vi "niDTS WLAN Rx Test Example.vi"() -> ()   [LabVIEW 2014]
uses:
  Includes/niDTS WLAN INC Type.ctl
  Rx Test/Includes/niDTS WLAN Rx Test INC Results.ctl
  CommLib/Includes/niDTS Comm INC EXE Port Parameters.ctl
  CommLib/Includes/niDTS Comm INC Telnet Port Parameters.ctl
  CommLib/Includes/niDTS Comm INC CLI Login.ctl
  HT Rx Test/Includes/niDTS WLAN HT Rx Test INC HT Parameters.ctl
  Includes/niDTS WLAN INC CH BW HT.ctl
  Includes/niDTS WLAN INC GI.ctl
  Includes/niDTS WLAN INC FEC Coding.ctl
  Rx Test/Includes/niDTS WLAN INC RX Measurement Parameters.ctl
  VHT Rx Test/Includes/niDTS WLAN VHT Rx Test INC Parameters.ctl
  Includes/niDTS WLAN INC CH BW.ctl
  OFDM Rx Test/Includes/niDTS WLAN Rx Test INC OFDM Parameters.ctl
  Includes/niDTS WLAN INC OFDM Data Rate.ctl
  Includes/niDTS WLAN INC CH BW DSSS.ctl
  TestStand/Station/Objects/SystemDutHandle/niDTS SystemDutHandle.lvclass
  niDTS WLAN.lvlib
  Plugins/niBCM4350/niBCM4350.lvlib
  Framework/niDTS Framework.lvlib
  TestStand/niDTS TestStand.lvlib
  Plugins/niBCM4360/niBCM4360.lvlib
  CommLib/niDTS CommLib.lvlib
  Plugins/niBCM4356/niBCM4356.lvlib
panel:
  in  "Socket Index":i32
  in  "System Configuration XML Path":path=path "C:/Users/Public/Documents/National Instruments/WTM 1.0/System Configurations"
  in  "Hardware Manifest XML":path=path "C:/Users/Public/Documents/National Instruments/WTM 1.0/Hardware Manifests"
  in  "Tab Control":enum32{"OFDM", "HT", "VHT"}(tab)=enum."HT"
  in  "OFDM Parameters":T1={"OFDM Data Rate (Mbps)"=enum."54", "Chains"=[TRUE, FALSE, FALSE, FALSE], "Bandwidth (Hz)"=enum."20 MHz", "Channel"=36, "Power (dBm)"=-50.0, "16 symbols"=TRUE, "Payload Length (bytes)"=1500, "Idle Interval (s)"=0.0001, "External Attenuation (dB)"=[2.0, 0.0, 0.0, 0.0], "RX Measurement Parameters"={"Number of Packets"=1000, "MacAddress"="FF:FF:FF:FF:FF:FF"}} {"Idle Interval (s)" format="%_3p"}
  in  "HT Parameters":T5={"MCS Index"=7, "Chains"=[TRUE, FALSE, FALSE, FALSE], "Bandwidth (Hz)"=enum."20 MHz", "Channel"=36, "Power (dBm)"=-45.0, "Guard Interval"=enum."LONG", "FEC Coding"=enum."LDPC", "16 symbols"=TRUE, "Payload Length (bytes)"=1500, "Idle Interval (s)"=5e-05, "External Attenuation (dB)"=[0.0, 0.0, 0.0, 0.0], "RX Measurement Parameters"={"Number of Packets"=1000, "MacAddress"="FF:FF:FF:FF:FF:FF"}} {"Idle Interval (s)" format="%_3p"}
  in  "VHT Parameters":T9={"MCS Index"=7, "N Spatial Streams"=1, "Chains"=[TRUE, FALSE, FALSE, FALSE], "Bandwidth (Hz)"=enum."20 MHz", "Channel"=36, "Power (dBm)"=-45.0, "Guard Interval"=enum."LONG", "FEC Coding"=enum."LDPC", "16 symbols"=TRUE, "Payload Length (bytes)"=1500, "Idle Interval (s)"=2.5e-05, "External Attenuation (dB)"=[0.0, 0.0, 0.0, 0.0], "RX Measurement Parameters"={"Number of Packets"=1000, "MacAddress"="FF:FF:FF:FF:FF:FF"}} {"Idle Interval (s)" format="%_3p"}
  out "error out":errorcluster
  in  "DUT Plugin":enum32{"BCM4360", "BCM4350", "BCM4356"}(tab)=enum."BCM4356"
  in  "Interfaces BCM4350":enum32{".EXE", "Telnet"}(tab)
  in  "General Parameters bcm4350 exe":T12={"WLAN"={"Port Parameters EXE"={"Timeout (s)"=5.0}}} caption="General Parameters"
  in  "Socket Parameters bcm4350 exe":cluster{"WLAN":cluster{"IP Address":string}}={"WLAN"={"IP Address"="192.168.1.1"}} caption="Socket Parameters"
  in  "Socket Parameters bcm4350 telnet":cluster{"WLAN":cluster{"IP Address":string}}={"WLAN"={"IP Address"="192.168.1.1"}} caption="Socket Parameters"
  in  "General Parameters bcm4350 telnet":T15={"WLAN"={"Port Parameters Telnet"={"Bytes to Read"=1000, "Line Separator"="\n", "Port Timeout (ms)"=5000, "Read Mode"=enum."normal", "Write Mode"=enum."normal", "Remote Port"=23}, "CLI Login"={"Do Login"=FALSE, "Login Prompt"="", "Password"="", "User Name"=""}}} caption="General Parameters"
  in  "General Parameters 4":T15={"WLAN"={"Port Parameters Telnet"={"Bytes to Read"=1000, "Line Separator"="\n", "Port Timeout (ms)"=5000, "Read Mode"=enum."normal", "Write Mode"=enum."normal", "Remote Port"=23}, "CLI Login"={"Do Login"=TRUE, "Login Prompt"="localhost login: ", "Password"="labview", "User Name"="root"}}} caption="General Parameters"
  in  "Socket Parameters bcm4356":cluster{"WLAN":cluster{"IP Address":string}}[](array[cluster])=[{"WLAN"={"IP Address"="192.168.0.31"}}, {"WLAN"={"IP Address"="192.168.0.32"}}, {"WLAN"={"IP Address"="192.168.0.33"}}, {"WLAN"={"IP Address"="192.168.0.34"}}] caption="Socket Parameters"
  out "Resutls":T16={"Packets Received"=1000, "PER (%)"=0.0}
  out "WLAN Type":T17=enum."n - MCS7"
  # "No Options"
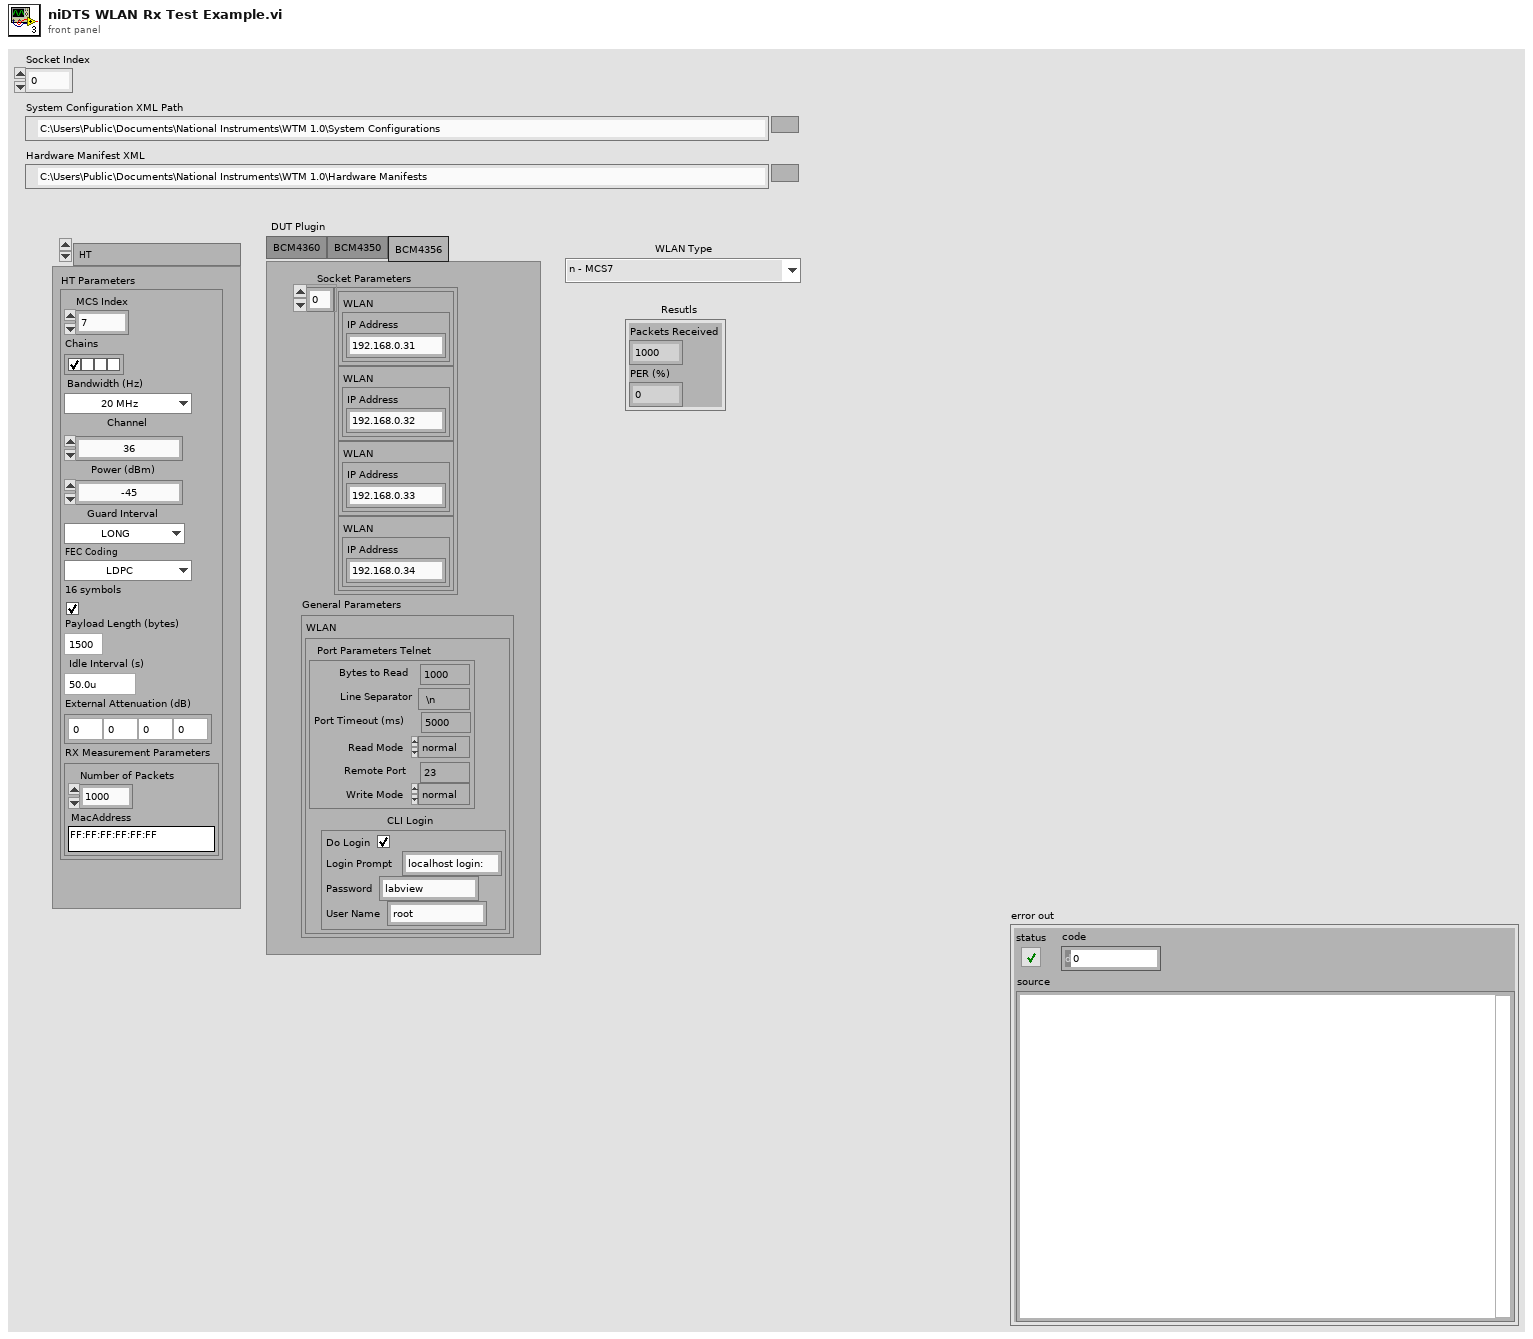
[diagram p1: front panel]
types:
  T1 = typedef "niDTS WLAN.lvlib/niDTS WLAN Rx Test INC OFDM Parameters.ctl" = cluster{"OFDM Data Rate (Mbps)":T2, "Chains":bool[], "Bandwidth (Hz)":T3, "Channel":i32, "Power (dBm)":dbl, "16 symbols":bool, "Payload Length (bytes)":i32, "Idle Interval (s)":dbl, "External Attenuation (dB)":dbl[], "RX Measurement Parameters":T4}
  T2 = typedef "niDTS WLAN.lvlib/niDTS WLAN INC OFDM Data Rate.ctl" = enum16{"6", "9", "12", "18", "24", "36", "48", "54"}
  T3 = typedef "niDTS WLAN.lvlib/niDTS WLAN INC CH BW DSSS.ctl" = enum16{"20 MHz"}
  T4 = typedef "niDTS WLAN.lvlib/niDTS WLAN INC RX Measurement Parameters.ctl" = cluster{"Number of Packets":i32, "MacAddress":string}
  T5 = typedef "niDTS WLAN.lvlib/niDTS WLAN HT Rx Test INC HT Parameters.ctl" = cluster{"MCS Index":i32, "Chains":bool[], "Bandwidth (Hz)":T6, "Channel":i32, "Power (dBm)":dbl, "Guard Interval":T7, "FEC Coding":T8, "16 symbols":bool, "Payload Length (bytes)":i32, "Idle Interval (s)":dbl, "External Attenuation (dB)":dbl[], "RX Measurement Parameters":T4}
  T6 = typedef "niDTS WLAN.lvlib/niDTS WLAN INC CH BW HT.ctl" = enum16{"20 MHz", "40 MHz"}
  T7 = typedef "niDTS WLAN.lvlib/niDTS WLAN INC GI.ctl" = enum16{"LONG", "SHORT"}
  T8 = typedef "niDTS WLAN.lvlib/niDTS WLAN INC FEC Coding.ctl" = enum16{"BCC", "LDPC"}
  T9 = typedef "niDTS WLAN.lvlib/niDTS WLAN VHT Rx Test INC Parameters.ctl" = cluster{"MCS Index":i32, "N Spatial Streams":i32, "Chains":bool[], "Bandwidth (Hz)":T10, "Channel":i32, "Power (dBm)":dbl, "Guard Interval":T7, "FEC Coding":T8, "16 symbols":bool, "Payload Length (bytes)":i32, "Idle Interval (s)":dbl, "External Attenuation (dB)":dbl[], "RX Measurement Parameters":T4}
  T10 = typedef "niDTS WLAN.lvlib/niDTS WLAN INC CH BW.ctl" = enum16{"20 MHz", "40 MHz", "80 MHz", "160 MHz"}
  T11 = typedef "niDTS CommLib.lvlib/niDTS Comm INC EXE Port Parameters.ctl" = cluster{"Timeout (s)":dbl}
  T12 = cluster{"WLAN":cluster{"Port Parameters EXE":T11}}
  T13 = typedef "niDTS CommLib.lvlib/niDTS Comm INC Telnet Port Parameters.ctl" = cluster{"Bytes to Read":i32, "Line Separator":string, "Port Timeout (ms)":i32, "Read Mode":enum16{"normal", "line", "buffered"}, "Write Mode":enum16{"normal", "line", "buffered"}, "Remote Port":u16}
  T14 = typedef "niDTS CommLib.lvlib/niDTS Comm INC CLI Login.ctl" = cluster{"Do Login":bool, "Login Prompt":string, "Password":string, "User Name":string}
  T15 = cluster{"WLAN":cluster{"Port Parameters Telnet":T13, "CLI Login":T14}}
  T16 = typedef "niDTS WLAN.lvlib/niDTS WLAN Rx Test INC Results.ctl" = cluster{"Packets Received":i32, "PER (%)":dbl}
  T17 = typedef "niDTS WLAN.lvlib/niDTS WLAN INC Type.ctl" = enum16{"b - 1 Mbps", "b - 2 Mbps", "b - 5.5 Mbps", "b - 11 Mbps", "ag - 6 Mbps", "ag - 9 Mbps", "ag - 12 Mbps", "ag - 18 Mbps", "ag - 24 Mbps", "ag - 36 Mbps", "ag - 48 Mbps", "ag - 54 Mbps", "n - MCS0", "n - MCS1", "n - MCS2", "n - MCS3", "n - MCS4", "n - MCS5", "n - MCS6", "n - MCS7", "n - MCS8", "n - MCS9", "n - MCS10", "n - MCS11", "n - MCS12", "n - MCS13", "n - MCS14", "n - MCS15", "n - MCS16", "n - MCS17", "n - MCS18", "n - MCS19", "n - MCS20", "n - MCS21", "n - MCS22", "n - MCS23", "n - MCS24", "n - MCS25", "n - MCS26", "n - MCS27", "n - MCS28", "n - MCS29", "n - MCS30", "n - MCS31", "ac - MCS0 -1", "ac - MCS1 -1", "ac - MCS2 -1", "ac - MCS3 -1", "ac - MCS4 -1", "ac - MCS5 -1", "ac - MCS6 -1", "ac - MCS7 -1", "ac - MCS8 -1", "ac - MCS9 -1", "ac - MCS0 -2", "ac - MCS1 -2", "ac - MCS2 -2", "ac - MCS3 -2", "ac - MCS4 -2", "ac - MCS5 -2", "ac - MCS6 -2", "ac - MCS7 -2", "ac - MCS8 -2", "ac - MCS9 -2", "ac - MCS0 -3", "ac - MCS1 -3", "ac - MCS2 -3", "ac - MCS3 -3", "ac - MCS4 -3", "ac - MCS5 -3", "ac - MCS6 -3", "ac - MCS7 -3", "ac - MCS8 -3", "ac - MCS9 -3", "ac - MCS0 -4", "ac - MCS1 -4", "ac - MCS2 -4", "ac - MCS3 -4", "ac - MCS4 -4", "ac - MCS5 -4", "ac - MCS6 -4", "ac - MCS7 -4", "ac - MCS8 -4", "ac - MCS9 -4"}
  T18 = typedef "niDTS Framework.lvlib/niDTS Logger INC Handle.ctl" = refnum<data-value>
  T19 = typedef "niDTS TestStand.lvlib/niDTS SystemDutHandle.lvclass/niDTS SystemDutHandle INC SystemDutHandles.ctl" = refnum<class "niDTS SystemDutHandle.lvclass">[]
  T20 = typedef "niDTS Framework.lvlib/niDTS Dut INC Handle.ctl" = refnum<data-value>
  T21 = typedef "niDTS WLAN.lvlib/niDTS WLAN Rx Test INC Handle.ctl" = refnum<data-value>
  T22 = typedef "niDTS WLAN.lvlib/niDTS WLAN Rx Test INC Parameters.ctl" = cluster{"Standard":T23, "DSSS Data Rate (Mbps)":T24, "OFDM Data Rate (Mbps)":T2, "MCS Index":i32, "N Spatial Streams":i32, "Chains":bool[], "Bandwidth (Hz)":T10, "Channel":i32, "Power (dBm)":dbl, "Guard Interval":T7, "FEC Coding":T8, "16 symbols":bool, "Payload Length (bytes)":i32, "Idle Interval (s)":dbl, "External Attenuation (dB)":dbl[], "RX Measurement Parameters":T4}
  T23 = typedef "niDTS WLAN.lvlib/niDTS WLAN INC Standard.ctl" = enum16{"802.11 b DSSS", "802.11 a/g OFDM", "802.11 n HT", "802.11 ac VHT"}
  T24 = typedef "niDTS WLAN.lvlib/niDTS WLAN INC DSSS Data Rate.ctl" = enum16{"1", "2", "5.5", "11"}
  T25 = typedef "niDTS WLAN.lvlib/niDTS WLAN DUT INC Parameters.ctl" = cluster{"WLAN Type":T17, "Bandwidth (Hz)":T10, "Channel":i32, "Guard Interval":T7, "FEC Coding":T8, "Power (dBm)":dbl, "Payload Length (bytes)":i32, "16 Symbols":bool, "Chains":bool[]}
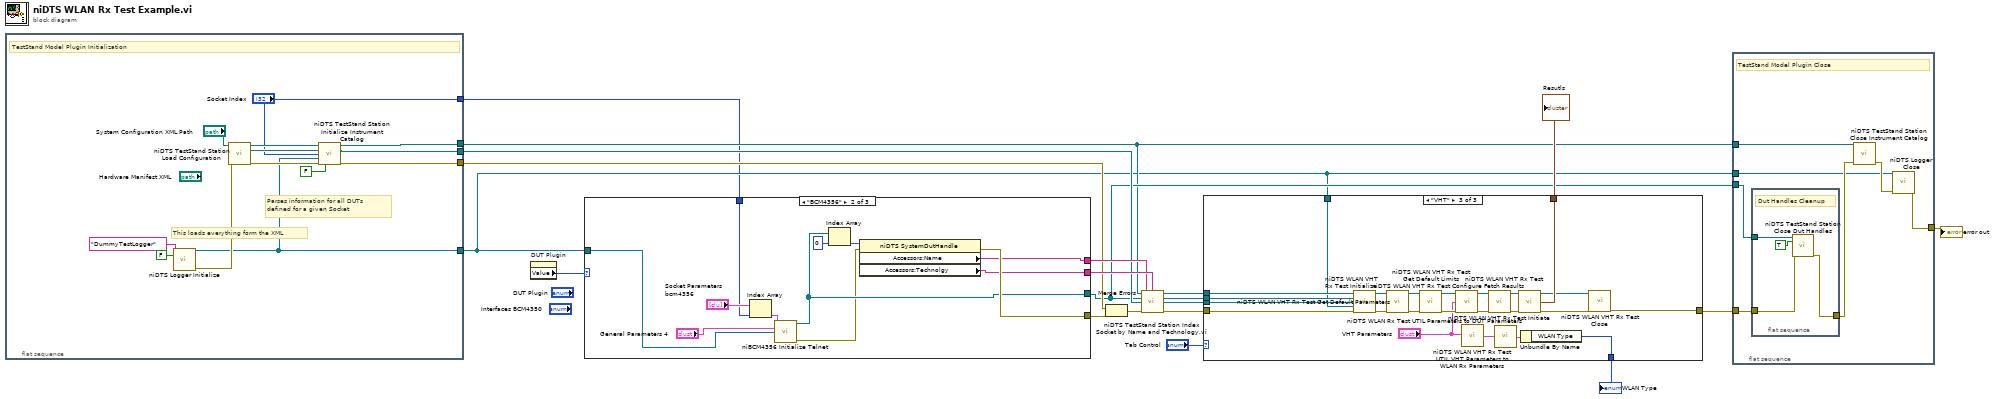
[diagram p0: block diagram]
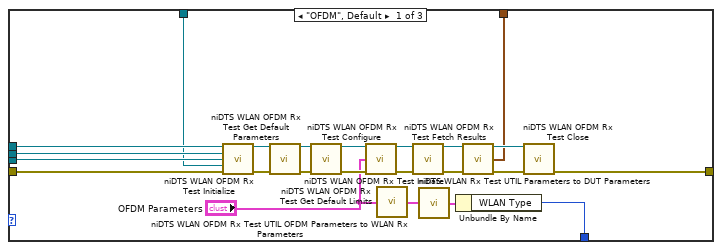
[diagram p2: hidden frame]
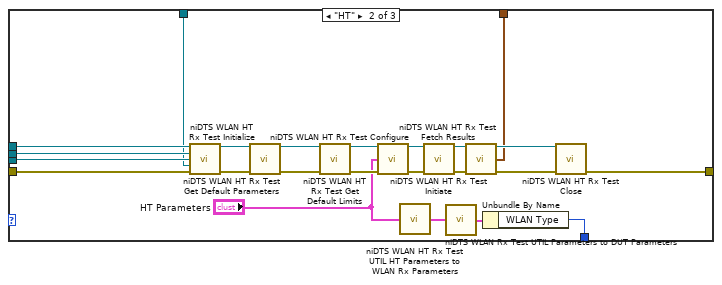
[diagram p3: hidden frame]
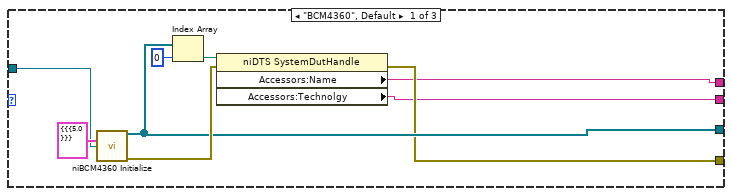
[diagram p4: hidden frame]
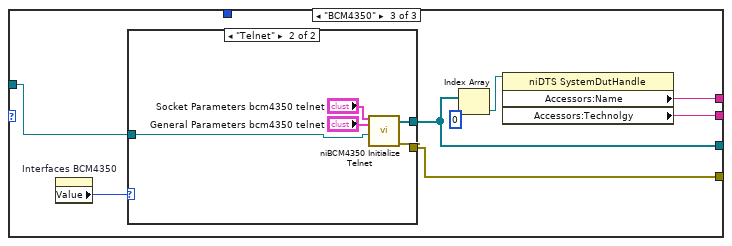
[diagram p5: hidden frame]
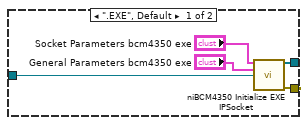
[diagram p6: hidden frame]
diagram:
  n1 = flat-sequence {
    tunnel: [w25] -> w12
    tunnel: [w26] -> w3
    tunnel: [w24] -> w13
    tunnel: [w23] -> w2
    tunnel: ["Socket Index"] -> w1
    frame #0 {
      # "Parses information for all DUTs defined for a given Socket"
      # "This loads everything form the XML"
      # "TestStand Model Plugin Initialization"
      n2 = call "niDTS Logger Initialize.vi"("Session Name ()"="DummyTestLogger", "Log to File"=FALSE) -> ("Logger Handle out"=w23:T18, "error out"=w30:errorcluster)  [unwired: 12 in]
      n3 = call "niDTS TestStand Station Load Configuration.vi"("System Configuration XML Path"="System Configuration XML Path", "error in (no error)"=w30) -> ("All System Hardware"=w27:refnum<class "niDTS SystemHardware.lvclass">, "All DUT Definitions"=w31:refnum<class "niDTS SystemDut.lvclass">[], "error out"=w28:errorcluster)  [unwired: 11 in]
      n4 = call "niDTS TestStand Station Initialize Instrument Catalog.vi"("All System Hardware"=w27, "All DUT Definitions"=w31, "Socket Index"="Socket Index", "Logger Handle"=w23, "error in (no error)"=w28, "Simulation Mode (F)"=FALSE) -> ("Socket Instrument Catalog"=w26:refnum<class "niDTS SystemInstrCatalog.lvclass">, "Socket DUT Definitions"=w25:refnum<class "niDTS SystemDut.lvclass">[], "error out"=w24:errorcluster)  [unwired: 7 in]
    }
  }
  n5 = property on="DUT Plugin" class="TabCtl (strict)"() -> ("Value"=w20:enum32{"BCM4360", "BCM4350", "BCM4356"})  [unwired: 2 in, 2 out]
  n6 = case shown="\"BCM4356\"" w20 {
    tunnel: [w37 w52 w58] -> w16
    tunnel: [w38 w47 w59] -> w4
    tunnel: w2 -> [w36 w48 w55]
    tunnel: [w35 w51 w57] -> w14
    tunnel: [w34 w50 w56] -> w15
    tunnel: w1 -> [_ w44 _]
    frame "BCM4360", Default {
      n7 = call "niBCM4360 Initialize.vi"("General Parameters"=T12 {"WLAN"={"Port Parameters EXE"={"Timeout (s)"=5.0}}}, "Logger"=w36) -> ("Dut Technology Handles"=w38:T19, "error out"=w42:errorcluster)  [unwired: 12 in]
      n8 = Index Array(array=w38, index=0) -> (element=w41:refnum<class "niDTS SystemDutHandle.lvclass">)
      n9 = property class="niDTS SystemDutHandle"(reference=w41, error in=w42) -> (error out=w37:errorcluster, "Accessors:Name"=w35:string, "Accessors:Technolgy"=w34:string)  [unwired: 1 out]
    }
    frame "BCM4356" {
      n10 = Index Array(array="Socket Parameters bcm4356", index=w44) -> (element=w43:cluster{"WLAN":cluster{"IP Address":string}})
      n11 = call "niBCM4356 Initialize Telnet.vi"("Socket Parameters"=w43, "General Parameters"="General Parameters 4", "Logger"=w48) -> ("Dut Technology Handles"=w47:T19, "error out"=w46:errorcluster)  [unwired: 11 in]
      n12 = Index Array(array=w47, index=0) -> (element=w54:refnum<class "niDTS SystemDutHandle.lvclass">)
      n13 = property class="niDTS SystemDutHandle"(reference=w54, error in=w46) -> (error out=w52:errorcluster, "Accessors:Name"=w51:string, "Accessors:Technolgy"=w50:string)  [unwired: 1 out]
    }
    frame "BCM4350" {
      n14 = property on="Interfaces BCM4350" class="TabCtl (strict)"() -> ("Value"=w62:enum32{".EXE", "Telnet"})  [unwired: 2 in, 2 out]
      n15 = case shown="\"Telnet\"" w62 {
        tunnel: [w66 w72] -> w58
        tunnel: [w67 w71] -> w59
        tunnel: w55 -> [w63 w68]
        frame ".EXE", Default {
          n16 = call "niBCM4350 Initialize EXE IPSocket.vi"("Socket Parameters"="Socket Parameters bcm4350 exe", "General Parameters"="General Parameters bcm4350 exe", "Logger"=w63) -> ("Dut Technology Handles 2"=w67:T19, "error out"=w66:errorcluster)  [unwired: 11 in]
        }
        frame "Telnet" {
          n17 = call "niBCM4350 Initialize Telnet.vi"("Socket Parameters"="Socket Parameters bcm4350 telnet", "General Parameters"="General Parameters bcm4350 telnet", "Logger"=w68) -> ("Dut Technology Handles"=w71:T19, "error out"=w72:errorcluster)  [unwired: 11 in]
        }
      }
      n18 = Index Array(array=w59, index=0) -> (element=w61:refnum<class "niDTS SystemDutHandle.lvclass">)
      n19 = property class="niDTS SystemDutHandle"(reference=w61) -> ("Accessors:Name"=w57:string, "Accessors:Technolgy"=w56:string)  [unwired: 1 in, 2 out]
    }
  }
  n20 = Merge Errors(w13, w16) -> (w17:errorcluster)
  n21 = call "niDTS TestStand Station Index Socket by Name and Technology,vi.vi"("niDTS SystemInstrCatalog in"=w3, "Name"=w14, "Technology"=w15, "System Dut Handles"=w4, "Socket DUT Definitions"=w12, "error in (no error)"=w17) -> ("Dut Handle"=w7:T20, "SystemTechnologyCatalog"=w8:refnum<class "niDTS SystemTechnologyCatalog.lvclass">, "Specific Socket/Tech DUT Definition"=w9:refnum<class "niDTS SystemDut.lvclass">, "error out"=w10:errorcluster)  [unwired: 6 in]
  n22 = case shown="\"VHT\"" "Tab Control" {
    tunnel: [w73 w118 w119] -> w18
    tunnel: w10 -> [w82 w104 w129]
    tunnel: w9 -> [w81 w103 w124]
    tunnel: w8 -> [w80 w102 w125]
    tunnel: w7 -> [w79 w101 w126]
    tunnel: w2 -> [w78 w100 w123]
    tunnel: [w83 w97 w130] -> w6
    tunnel: [w74 w96 w131] -> w5
    frame "OFDM", Default {
      n23 = call "niDTS WLAN OFDM Rx Test Initialize.vi"("Dut Reference"=w79, "SystemTechnologyCatalog"=w80, "SystemDut"=w81, "Logger Reference"=w78, "error in (no error)"=w82) -> ("Dummy Test Handle out"=w90:T21, "error out"=w89:errorcluster)  [unwired: 8 in, 1 out]
      n24 = call "niDTS WLAN OFDM Rx Test Get Default Parameters.vi"("Dummy Test Handle in"=w90, "error in (no error)"=w89) -> ("Dummy Test Handle out"=w85:T21, "error out"=w84:errorcluster)  [unwired: 11 in, 1 out]
      n25 = call "niDTS WLAN OFDM Rx Test Get Default Limits.vi"("Dummy Test Handle in"=w85, "error in (no error)"=w84) -> ("Dummy Test Handle out"=w88:T21, "error out"=w87:errorcluster)  [unwired: 10 in, 2 out]
      n26 = call "niDTS WLAN OFDM Rx Test Configure.vi"("Dummy Test Handle in"=w88, "WLAN Rx Input Parameters"="OFDM Parameters", "error in (no error)"=w87) -> ("Dummy Test Handle out"=w95:T21, "error out"=w86:errorcluster)  [unwired: 11 in]
      n27 = call "niDTS WLAN OFDM Rx Test UTIL OFDM Parameters to WLAN Rx Parameters.vi"("WLAN Rx Input Parameters"="OFDM Parameters") -> ("WLAN Tx Parameters"=w77:T22)  [unwired: 14 in]
      n28 = call "niDTS WLAN OFDM Rx Test Initiate.vi"("Dummy Test Handle in"=w95, "error in (no error)"=w86) -> ("Dummy Test Handle out"=w94:T21, "error out"=w93:errorcluster)  [unwired: 12 in]
      n29 = call "niDTS WLAN Rx Test UTIL Parameters to DUT Parameters.vi"("Parameters"=w77) -> ("TV Parameters(DataType)"=w76:T25)  [unwired: 14 in]
      n30 = Unbundle By Name(w76) -> ("WLAN Type"=w74:T17)
      n31 = call "niDTS WLAN OFDM Rx Test Fetch Results.vi"("Dummy Test Handle in"=w94, "error in (no error)"=w93) -> ("Dummy Test Handle out"=w92:T21, "Resutls"=w83:T16, "error out"=w91:errorcluster)  [unwired: 11 in]
      n32 = call "niDTS WLAN OFDM Rx Test Close.vi"("Dummy Test Handle in"=w92, "error in (no error)"=w91) -> ("error out"=w73:errorcluster)  [unwired: 13 in]
    }
    frame "HT" {
      n33 = call "niDTS WLAN HT Rx Test Initialize.vi"("Dut Reference"=w101, "SystemTechnologyCatalog"=w102, "SystemDut"=w103, "Logger Reference"=w100, "error in (no error)"=w104) -> ("Dummy Test Handle out"=w111:T21, "error out"=w110:errorcluster)  [unwired: 8 in, 1 out]
      n34 = call "niDTS WLAN HT Rx Test Get Default Parameters.vi"("Dummy Test Handle in"=w111, "error in (no error)"=w110) -> ("Dummy Test Handle out"=w106:T21, "error out"=w105:errorcluster)  [unwired: 11 in, 1 out]
      n35 = call "niDTS WLAN HT Rx Test Get Default Limits.vi"("Dummy Test Handle in"=w106, "error in (no error)"=w105) -> ("Dummy Test Handle out"=w109:T21, "error out"=w108:errorcluster)  [unwired: 10 in, 2 out]
      n36 = call "niDTS WLAN HT Rx Test Configure.vi"("Dummy Test Handle in"=w109, "WLAN HT Rx Input Parameters"="HT Parameters", "error in (no error)"=w108) -> ("Dummy Test Handle out"=w116:T21, "error out"=w107:errorcluster)  [unwired: 11 in]
      n37 = call "niDTS WLAN HT Rx Test UTIL HT Parameters to WLAN Rx Parameters.vi"("HT Rx Input Parameters"="HT Parameters") -> ("WLAN Tx Parameters"=w98:T22)  [unwired: 14 in]
      n38 = call "niDTS WLAN HT Rx Test Initiate.vi"("Dummy Test Handle in"=w116, "error in (no error)"=w107) -> ("Dummy Test Handle out"=w115:T21, "error out"=w114:errorcluster)  [unwired: 12 in]
      n39 = call "niDTS WLAN Rx Test UTIL Parameters to DUT Parameters.vi"("Parameters"=w98) -> ("TV Parameters(DataType)"=w117:T25)  [unwired: 14 in]
      n40 = call "niDTS WLAN HT Rx Test Fetch Results.vi"("Dummy Test Handle in"=w115, "error in (no error)"=w114) -> ("Dummy Test Handle out"=w113:T21, "Resutls"=w97:T16, "error out"=w112:errorcluster)  [unwired: 11 in]
      n41 = Unbundle By Name(w117) -> ("WLAN Type"=w96:T17)
      n42 = call "niDTS WLAN HT Rx Test Close.vi"("Dummy Test Handle in"=w113, "error in (no error)"=w112) -> ("error out"=w118:errorcluster)  [unwired: 13 in]
    }
    frame "VHT" {
      n43 = call "niDTS WLAN VHT Rx Test Initialize.vi"("Dut Reference"=w126, "SystemTechnologyCatalog"=w125, "SystemDut"=w124, "Logger Reference"=w123, "error in (no error)"=w129) -> ("Dummy Test Handle out"=w138:T21, "error out"=w137:errorcluster)  [unwired: 8 in, 1 out]
      n44 = call "niDTS WLAN VHT Rx Test Get Default Parameters.vi"("Dummy Test Handle in"=w138, "error in (no error)"=w137) -> ("Dummy Test Handle out"=w133:T21, "error out"=w132:errorcluster)  [unwired: 11 in, 1 out]
      n45 = call "niDTS WLAN VHT Rx Test Get Default Limits.vi"("Dummy Test Handle in"=w133, "error in (no error)"=w132) -> ("Dummy Test Handle out"=w136:T21, "error out"=w135:errorcluster)  [unwired: 10 in, 2 out]
      n46 = call "niDTS WLAN VHT Rx Test Configure.vi"("Dummy Test Handle in"=w136, "WLAN Rx Input Parameters"="VHT Parameters", "error in (no error)"=w135) -> ("Dummy Test Handle out"=w141:T21, "error out"=w134:errorcluster)  [unwired: 11 in]
      n47 = call "niDTS WLAN VHT Rx Test UTIL VHT Parameters to WLAN Rx Parameters.vi"("WLAN Rx Input Parameters"="VHT Parameters") -> ("WLAN Tx Parameters"=w127:T22)  [unwired: 14 in]
      n48 = call "niDTS WLAN VHT Rx Test Initiate.vi"("Dummy Test Handle in"=w141, "error in (no error)"=w134) -> ("Dummy Test Handle out"=w140:T21, "error out"=w139:errorcluster)  [unwired: 12 in]
      n49 = call "niDTS WLAN Rx Test UTIL Parameters to DUT Parameters.vi"("Parameters"=w127) -> ("TV Parameters(DataType)"=w122:T25)  [unwired: 14 in]
      n50 = call "niDTS WLAN VHT Rx Test Fetch Results.vi"("Dummy Test Handle in"=w140, "error in (no error)"=w139) -> ("Dummy Test Handle out"=w121:T21, "Resutls"=w130:T16, "error out"=w120:errorcluster)  [unwired: 11 in]
      n51 = Unbundle By Name(w122) -> ("WLAN Type"=w131:T17)
      n52 = call "niDTS WLAN VHT Rx Test Close.vi"("Dummy Test Handle in"=w121, "error in (no error)"=w120) -> ("error out"=w119:errorcluster)  [unwired: 13 in]
    }
  }
  "Resutls" <- w6
  "WLAN Type" <- w5
  n53 = flat-sequence {
    tunnel: [w148] -> w19
    tunnel: w18 -> [w147]
    tunnel: w4 -> [w146]
    tunnel: w3 -> [w143]
    tunnel: w2 -> [w142]
    frame #0 {
      # "TestStand Model Plugin Close"
      n54 = flat-sequence {
        tunnel: w147 -> [w151]
        tunnel: [w150] -> w145
        tunnel: w146 -> [w149]
        frame #0 {
          # "Dut Handles Cleanup"
          n55 = call "niDTS TestStand Station Close Dut Handles.vi"("Socket Dut Handles In"=w149, "Close All"=TRUE, "error in (no error)"=w151) -> ("error out"=w150:errorcluster)  [unwired: 11 in, 1 out]
        }
      }
      n56 = call "niDTS TestStand Station Close Instrument Catalog.vi"("Socket Instrument Catalog"=w143, "error in (no error)"=w145) -> ("error out"=w144:errorcluster)  [unwired: 13 in]
      n57 = call "niDTS Logger Close.vi"("Logger Handle in"=w142, "error in (no error)"=w144) -> ("error out"=w148:errorcluster)  [unwired: 13 in]
    }
  }
  "error out" <- w19
